vi "Smoother Controls.vi"(9 "Proportional Constant":dbl, 10 "New Input":dbl(slide) scale=-1.0..1.0, 11 "Previous Value":dbl format="%#_13g") -> (3 "Motor Setpoint":dbl(slide) scale=-1.0..1.0)   [LabVIEW 2018]
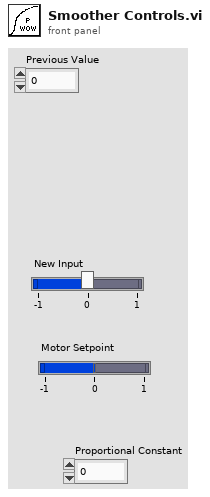
[diagram p1: front panel]
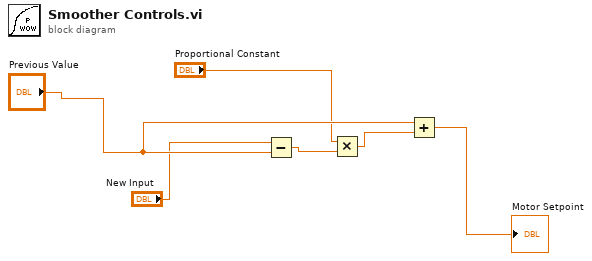
[diagram p0: block diagram]
diagram:
  n1 = Subtract(x="New Input", y="Previous Value") -> (x-y=w4:dbl)
  n2 = Multiply(x="Proportional Constant", y=w4) -> (x*y=w2:dbl)
  n3 = Add(x="Previous Value", y=w2) -> (x+y=→"Motor Setpoint":dbl)
